vi "Get and Set LED.vi"(9 "Display Mode":T1(ring), 10 "Color":T2(ring), 11 "refnum name":string="My LED refnum") -> ()   [LabVIEW 2016]
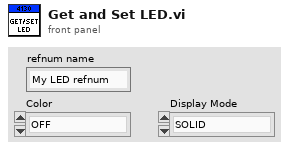
[diagram p1: front panel]
types:
  T1 = enum16{"SOLID", "FLASH 500ms", "FLASH 1000ms", "OFF"}
  T2 = enum16{"OFF", "RED", "GREEN", "BLUE", "PURPLE", "YELLOW", "TEAL", "WHITE", "RAINBOW"}
  T3 = typedef "WPI_DigitalOutputDevRef.ctl" = cluster{"DIO Channel":T4, "DevStatus":errorcluster}
  T4 = typedef "FPGA_DIOChannel.ctl" = enum8{"DIO 0", "DIO 1", "DIO 2", "DIO 3", "DIO 4", "DIO 5", "DIO 6", "DIO 7", "DIO 8", "DIO 9", "DIO MXP 0", "DIO MXP 1", "DIO MXP 2", "DIO MXP 3", "DIO MXP 4", "DIO MXP 5", "DIO MXP 6", "DIO MXP 7", "DIO MXP 8", "DIO MXP 9", "DIO MXP 10", "DIO MXP 11", "DIO MXP 12", "DIO MXP 13", "DIO MXP 14", "DIO MXP 15", "SPI Port CS1", "SPI Port CS2", "SPI Port CS3", "SPI Port MISO", "SPI Port MOSI", "Invalid"}
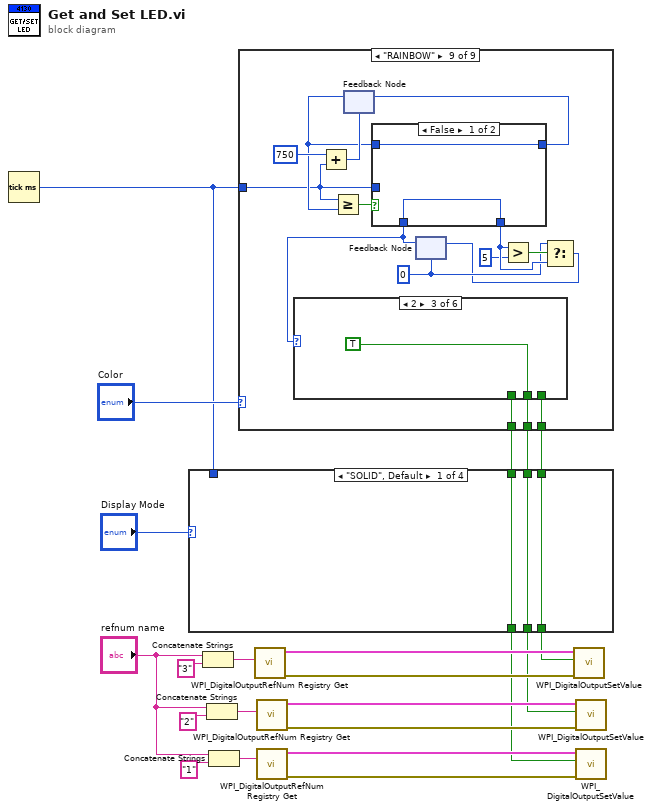
[diagram p0: block diagram]
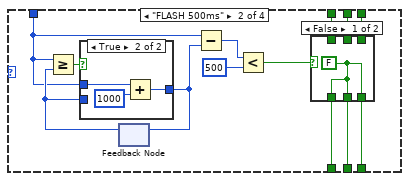
[diagram p2: hidden frame]
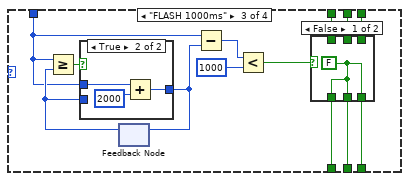
[diagram p5: hidden frame]
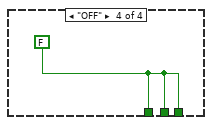
[diagram p8: hidden frame]
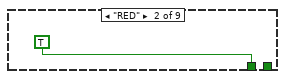
[diagram p10: hidden frame]
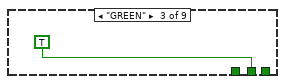
[diagram p11: hidden frame]
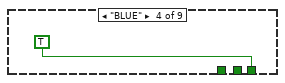
[diagram p12: hidden frame]
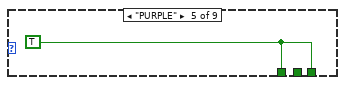
[diagram p13: hidden frame]
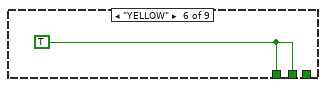
[diagram p14: hidden frame]
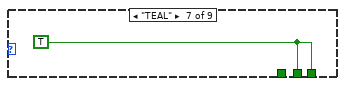
[diagram p15: hidden frame]
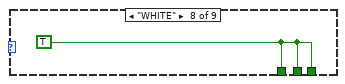
[diagram p16: hidden frame]
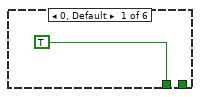
[diagram p17: hidden frame]
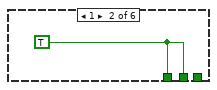
[diagram p18: hidden frame]
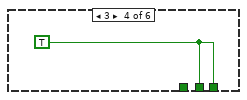
[diagram p19: hidden frame]
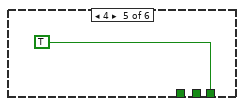
[diagram p20: hidden frame]
diagram:
  n1 = Tick Count (ms)() -> (millisecond timer value=w1:u32)
  n2 = Concatenate Strings("refnum name", "3" ("string")) -> (w18:string)
  n3 = Concatenate Strings("refnum name", "2" ("string")) -> (w19:string)
  n4 = Concatenate Strings("refnum name", "1" ("string")) -> (w20:string)
  n5 = case shown="\"RAINBOW\"" "Color" {
    tunnel: [_ _ _ TRUE w26 _ w28 w29 w32] -> w2
    tunnel: [_ _ TRUE _ _ w27 w28 w29 w31] -> w4
    tunnel: [_ TRUE _ _ w26 w27 _ w29 w33] -> w6
    tunnel: w1 -> [_ _ _ _ _ _ _ _ w30]
    frame "OFF", Default {
    }
    frame "RED" {
    }
    frame "GREEN" {
    }
    frame "BLUE" {
    }
    frame "PURPLE" {
      w26 = TRUE
    }
    frame "YELLOW" {
      w27 = TRUE
    }
    frame "TEAL" {
      w28 = TRUE
    }
    frame "WHITE" {
      w29 = TRUE
    }
    frame "RAINBOW" {
      w35 = 0
      n6 = Add(x=u32 750, y=w30) -> (x+y=w42:u32)
      n7 = feedback #1(w42) -> (w40:u32)
      n8 = Greater Or Equal?(x=w30, y=w40) -> (x >= y?=w41:bool)
      n9 = feedback #2(w35) -> (w39:i32)
      n10 = case shown="2" w39 {
        tunnel: [TRUE w46 _ _ _ w50] -> w33
        tunnel: [_ _ _ w48 TRUE w50] -> w32
        tunnel: [_ w46 TRUE w48 _ _] -> w31
        frame 0, Default {
        }
        frame 1 {
          w46 = TRUE
        }
        frame 2 {
        }
        frame 3 {
          w48 = TRUE
        }
        frame 4 {
        }
        frame 5 {
          w50 = TRUE
        }
      }
      n11 = case shown="False" w41 {
        tunnel: w30 -> [_ w57]
        tunnel: [w52 w55] -> w44
        tunnel: w40 -> [w52 _]
        tunnel: w39 -> [w51 w54]
        tunnel: [w51 w53] -> w37
        frame False {
        }
        frame True {
          n12 = Add(x=u32 333, y=w57) -> (x+y=w55:u32)
          n13 = Increment(x=w54) -> (x+1=w53:i32)
        }
      }
      n14 = feedback-in #1(w44) -> ()
      n15 = Greater?(x=w37, y=5) -> (0:w38:bool)
      n16 = Select(t=w35, s=w38, f=w37) -> (s? t:f=w34:i32)
      n17 = feedback-in #2(w34) -> ()
    }
  }
  n18 = case shown="\"SOLID\", Default" "Display Mode" {
    tunnel: [w60 w69 w90 w103] -> w7
    tunnel: w6 -> [w60 w68 w89 _]
    tunnel: [w59 w71 w92 w103] -> w5
    tunnel: w4 -> [w59 w70 w91 _]
    tunnel: [w58 w73 w94 w103] -> w3
    tunnel: w2 -> [w58 w72 w93 _]
    tunnel: w1 -> [_ w65 w86 _]
    frame "SOLID", Default {
    }
    frame "FLASH 500ms" {
      n19 = feedback #3() -> (w66:u32)  [unwired: 1 in]
      n20 = Greater Or Equal?(x=w65, y=w66) -> (x >= y?=w67:bool)
      n21 = case shown="True" w67 {
        tunnel: w65 -> [_ w77]
        tunnel: [w74 w76] -> w64
        tunnel: w66 -> [w74 _]
        frame False {
        }
        frame True {
          n22 = Add(x=w77, y=u32 1000) -> (x+y=w76:u32)
        }
      }
      n23 = feedback-in #3(w64) -> ()
      n24 = Subtract(x=w65, y=w64) -> (x-y=w63:u32)
      n25 = Less?(x=w63, y=u32 500) -> (x < y?=w61:bool)
      n26 = case shown="False" w61 {
        tunnel: [w78 w81] -> w73
        tunnel: w72 -> [_ w81]
        tunnel: [w78 w80] -> w71
        tunnel: w70 -> [_ w80]
        tunnel: [w78 w79] -> w69
        tunnel: w68 -> [_ w79]
        frame False {
          w78 = FALSE
        }
        frame True {
        }
      }
    }
    frame "FLASH 1000ms" {
      n27 = feedback #4() -> (w87:u32)  [unwired: 1 in]
      n28 = Greater Or Equal?(x=w86, y=w87) -> (x >= y?=w88:bool)
      n29 = case shown="True" w88 {
        tunnel: w86 -> [_ w98]
        tunnel: [w95 w97] -> w85
        tunnel: w87 -> [w95 _]
        frame False {
        }
        frame True {
          n30 = Add(x=w98, y=u32 2000) -> (x+y=w97:u32)
        }
      }
      n31 = feedback-in #4(w85) -> ()
      n32 = Subtract(x=w86, y=w85) -> (x-y=w84:u32)
      n33 = Less?(x=w84, y=u32 1000) -> (x < y?=w82:bool)
      n34 = case shown="False" w82 {
        tunnel: [w99 w102] -> w94
        tunnel: w93 -> [_ w102]
        tunnel: [w99 w101] -> w92
        tunnel: w91 -> [_ w101]
        tunnel: [w99 w100] -> w90
        tunnel: w89 -> [_ w100]
        frame False {
          w99 = FALSE
        }
        frame True {
        }
      }
    }
    frame "OFF" {
      w103 = FALSE
    }
  }
  n35 = call <vilib>:"WPI_DigitalOutputRefNum Registry Get.vi"("refnum name"=w18) -> ("error out"=w9:errorcluster, "DigitalOutputDevRef"=w10:T3)  [unwired: 9 in]
  n36 = call <vilib>:"WPI_DigitalOutputRefNum Registry Get.vi"("refnum name"=w19) -> ("error out"=w12:errorcluster, "DigitalOutputDevRef"=w11:T3)  [unwired: 9 in]
  n37 = call <vilib>:"WPI_DigitalOutputRefNum Registry Get.vi"("refnum name"=w20) -> ("error out"=w13:errorcluster, "DigitalOutputDevRef"=w14:T3)  [unwired: 9 in]
  n38 = call <vilib>:"WPI_DigitalOutputSetValue.vi"("error in (no error)"=w9, "Value"=w3, "DigitalOutputDevRef"=w10) -> ()  [unwired: 7 in, 2 out]
  n39 = call <vilib>:"WPI_DigitalOutputSetValue.vi"("error in (no error)"=w12, "Value"=w5, "DigitalOutputDevRef"=w11) -> ()  [unwired: 7 in, 2 out]
  n40 = call <vilib>:"WPI_DigitalOutputSetValue.vi"("error in (no error)"=w13, "Value"=w7, "DigitalOutputDevRef"=w14) -> ()  [unwired: 7 in, 2 out]
